vi "unwrapSequence.vi"(9 "result array in":dbl[][](array[numeric]), 10 "value in":dbl, 11 "index in":i32) -> (3 "result array out":dbl[][](array[numeric]))   [LabVIEW 2018, in "myFFT.lvlib"]
uses:
  myFFT.lvlib
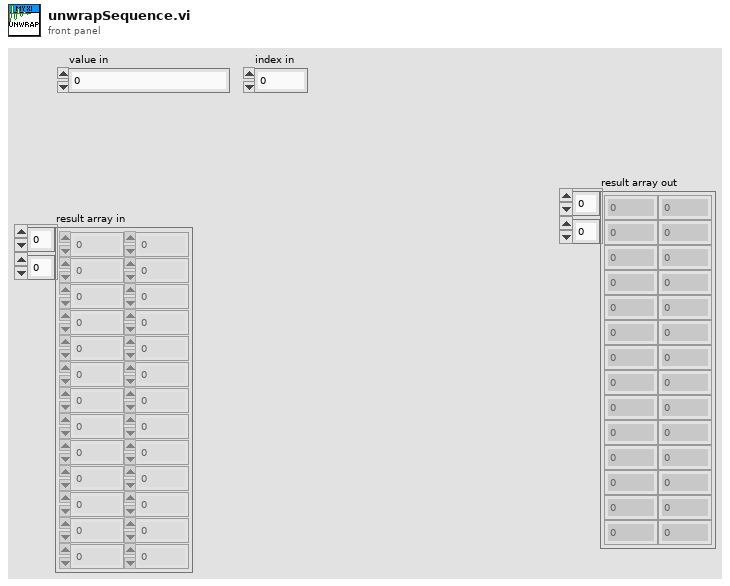
[diagram p1: front panel]
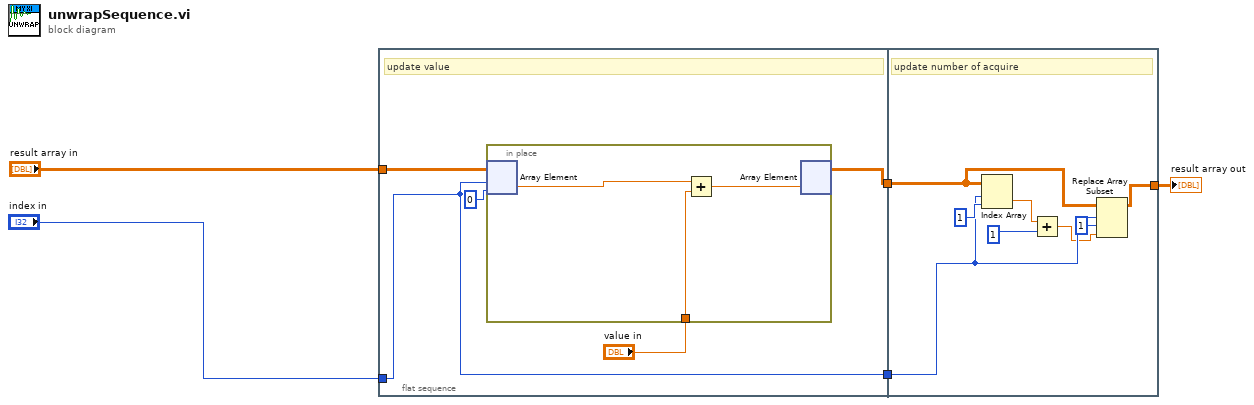
[diagram p0: block diagram]
diagram:
  n1 = flat-sequence {
    tunnel: "index in" -> [w9]
    tunnel: "result array in" -> [w10]
    tunnel: [w8] -> w3
    tunnel: [w9] -> w2
    tunnel: w3 -> [w18]
    tunnel: w2 -> [w16]
    tunnel: [w17] -> w1
    frame #0 {
      # "update value"
      n2 = in-place {
        in-place-border: "value in" -> [w13]
        n3 = in-place-array #1(w10, w9, 0) -> (w12:dbl)
        n4 = Add(x=w12, y=w13) -> (x+y=w11:dbl)
        n5 = in-place-array #1(w11) -> (w8:dbl[][])  [unwired: 2 out]
      }
    }
    frame #1 {
      # "update number of acquire"
      n6 = Index Array(array=w18, index (row)=w16, index (col)=1 ("disabled index (col)")) -> (element=w20:dbl)
      n7 = Add(x=w20, y=1) -> (x+y=w14:dbl)
      n8 = Replace Array Subset(array=w18, new element=w14, index (row)=w16, index (col)=1 ("disabled index (col)")) -> (w17:dbl[][])
    }
  }
  "result array out" <- w1
